vi "WriteCoils.vi"(3 "BEEP":bool, 4 "LED1":bool, 5 "LED0":bool) -> (2 "Coils to Write Ouput":bool[](array[boolean]))   [LabVIEW 2013]
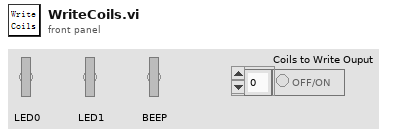
[diagram p1: front panel]
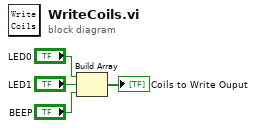
[diagram p0: block diagram]
diagram:
  n1 = Build Array("LED0", "LED1", "BEEP") -> (→"Coils to Write Ouput":bool[])
